vi "LockInSubVI.vi"(3 "error in":errorcluster, 4 "mode (0)":i16, 5 "address string":string="19") -> (0 "error out 2":errorcluster, 1 "data Y":dbl, 2 "data X":dbl)   [LabVIEW 2010]
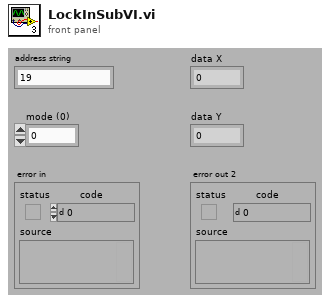
[diagram p1: front panel]
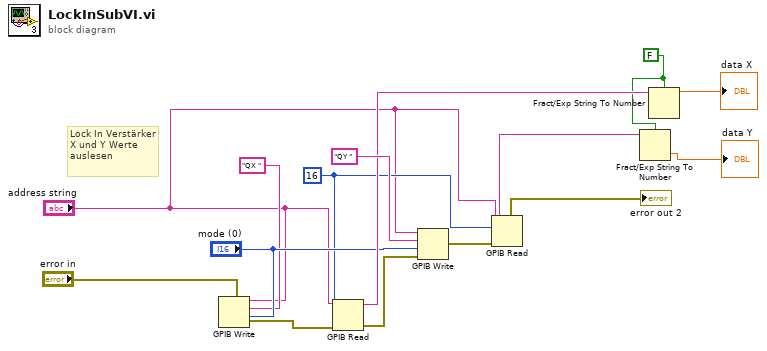
[diagram p0: block diagram]
diagram:
  w1 = FALSE
  w9 = 16
  # "Lock In Verstärker X und Y Werte auslesen"
  n1 = GPIB Write(0:"address string", 1:"QX ", 2:"mode (0)", 3:"error in") -> (6:w3:errorcluster)  [unwired: 1 in, 1 out]
  n2 = GPIB Read(0:"address string", 1:w9, 3:w3) -> (5:w12:string, 7:w4:errorcluster)  [unwired: 2 in, 1 out]
  n3 = GPIB Write(0:"address string", 1:"QY ", 2:"mode (0)", 3:w4) -> (6:w5:errorcluster)  [unwired: 1 in, 1 out]
  n4 = GPIB Read(0:"address string", 1:w9, 3:w5) -> (5:w11:string, 7:→"error out 2":errorcluster)  [unwired: 2 in, 1 out]
  n5 = Fract/Exp String To Number(use system decimal point (T)=w1, string=w11) -> (number=→"data Y":dbl)  [unwired: 2 in, 1 out]
  n6 = Fract/Exp String To Number(use system decimal point (T)=w1, string=w12) -> (number=→"data X":dbl)  [unwired: 2 in, 1 out]
